vi "MH_Ext_Acquire.vi"(8 "error in (no error)":errorcluster, 10 "event data":cluster{"Last Move?":bool, "First Move?":bool}, 11 "SinglePhotonInterferenceUI in":refnum<class "SinglePhotonInterferenceUI.lvclass">) -> (0 "error out":errorcluster, 3 "SinglePhotonInterferenceUI out":refnum<class "SinglePhotonInterferenceUI.lvclass">)   [LabVIEW 2023, in "SinglePhotonInterferenceUI.lvlib" / "SinglePhotonInterferenceUI.lvclass"]
uses:
  SinglePhotonInterferenceUI.lvclass
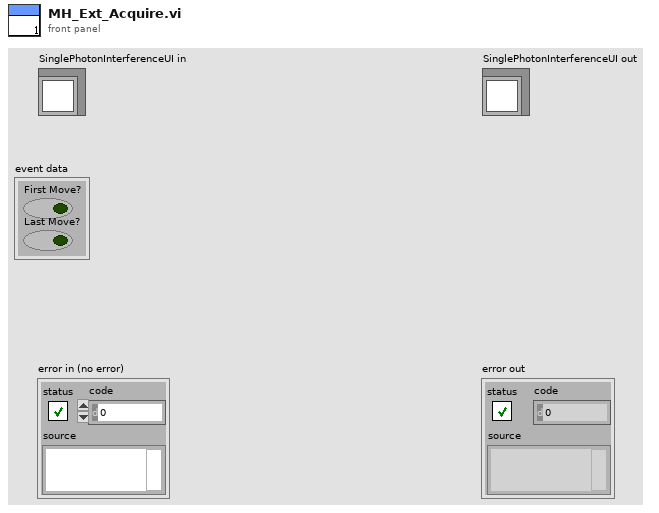
[diagram p1: front panel]
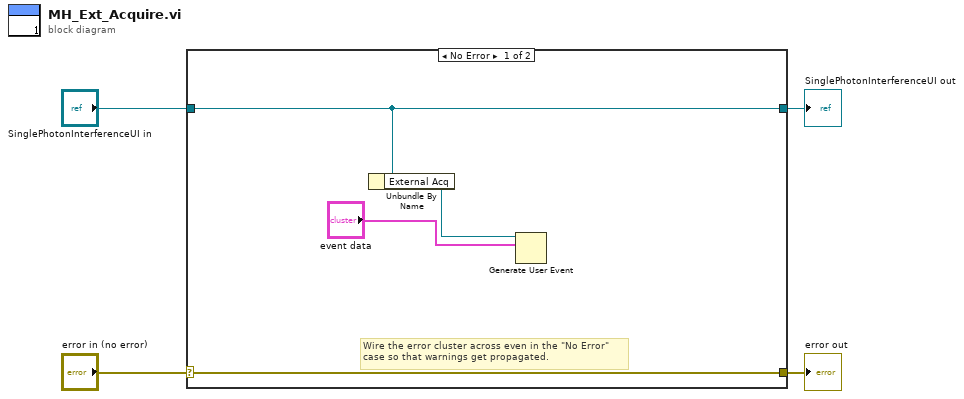
[diagram p0: block diagram]
diagram:
  n1 = case shown="No Error" "error in (no error)" {
    selector: "error in (no error)" -> [w8 w10]
    tunnel: [w8 w10] -> w3
    tunnel: [w7 w9] -> w1
    tunnel: "SinglePhotonInterferenceUI in" -> [w7 w9]
    frame No Error {
      # "Wire the error cluster across even in the \"No Error\"\ncase so that warnings get propagated."
      n2 = Unbundle By Name(w7) -> ("External Acq"=w6:refnum<user-event>)
      n3 = Generate User Event(user event=w6, event data cluster="event data") -> ()  [unwired: 2 in, 2 out]
    }
    frame Error {
    }
  }
  "error out" <- w3
  "SinglePhotonInterferenceUI out" <- w1
